vi "Metric To Prometheus Lines.vi"(8 "error in (no error)":errorcluster, 10 "Include Metadata":bool=TRUE, 11 "Counters.lvlib:Counter.lvclass":refnum<class "Counter.lvclass">) -> (0 "error out":errorcluster, 3 "Prometheus Lines":string[](array[string]))   [LabVIEW 2020, in "Metrics.lvlib" / "Counter.lvclass"]
uses:
  Counter.lvclass
  Counter.lvclass/Counter.ctl
  metric/Metric.lvclass
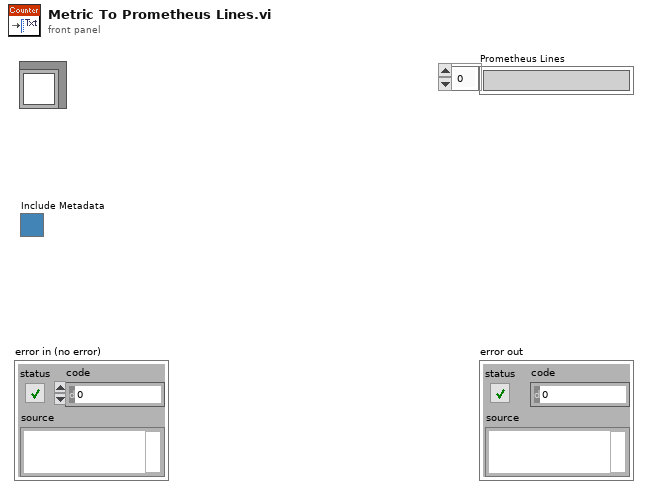
[diagram p1: front panel]
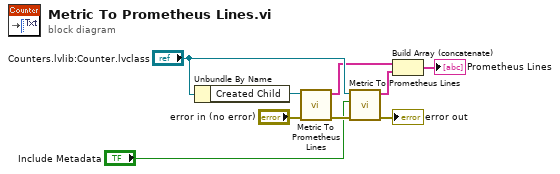
[diagram p0: block diagram]
diagram:
  n1 = Unbundle By Name("Counters.lvlib:Counter.lvclass") -> ("Created Child"=w7:refnum<class "Metric.lvclass">)
  n2 = call-dynamic "Metric To Prometheus Lines.vi"("error in (no error)"="error in (no error)", "Metrics.lvlib:Metric.lvclass"=w7) -> ("error out"=w2:errorcluster, "Prometheus Lines"=w6:string[])  [unwired: 8 in]
  n3 = call-parent "Metric To Prometheus Lines.vi"("error in (no error)"=w2, "Include Metadata"="Include Metadata", "Metrics.lvlib:Metric.lvclass"="Counters.lvlib:Counter.lvclass") -> ("error out"=→"error out":errorcluster, "Prometheus Lines"=w5:string[])  [unwired: 7 in]
  n4 = Build Array (concatenate)(w6, w5) -> (→"Prometheus Lines":string[])
